vi "FTW-Example-SLASD-Launch.vi"(9 "Timeout":i32=1000 format="%dmsec", 11 "error in":errorcluster) -> (4 "FTW Actor Connector":refnum<class "FTW-Example-SLASD.lvclass">, 6 "Initialized Response":string, 8 "Instance Inbox Address":string, 10 "Instance Publisher Address":string, 15 "error out":errorcluster)   [LabVIEW 2013]
uses:
  FTW-Example-SLASD.lvclass
  Actor/src/Connector/FTW-ActorConnector.lvclass
  Core/FTW-Example-SLASD-Core.lvclass
panel:
  in  "Boolean":bool
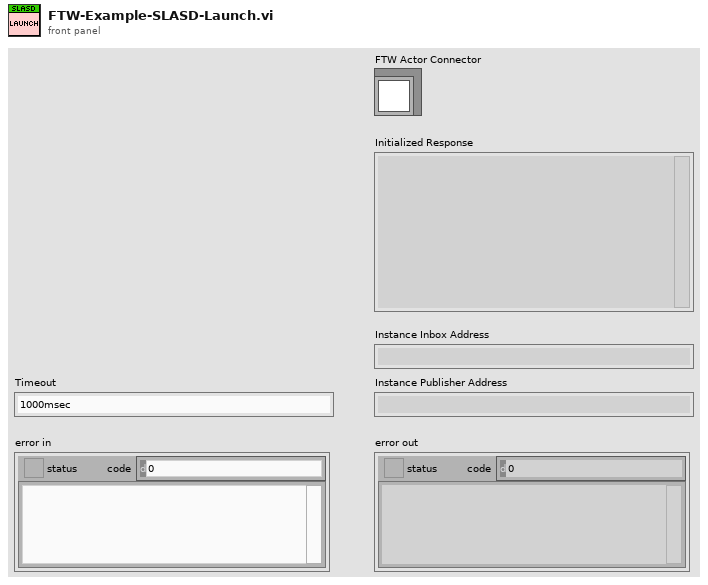
[diagram p1: front panel]
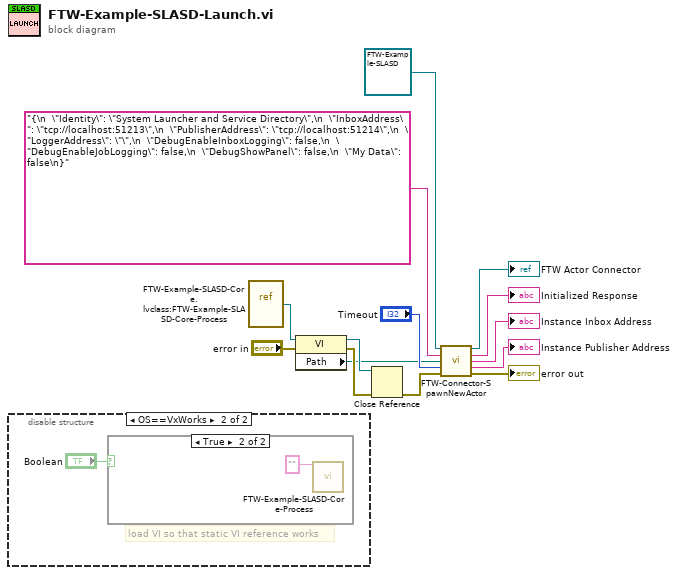
[diagram p0: block diagram]
diagram:
  n1 = disable-structure shown="OS==VxWorks" {
    frame condition #0 (active) {
    }
    frame condition #1 {
      # "load VI so that static VI reference works"
      n2 = case shown="True" "Boolean" {
        frame False {
        }
        frame True {
          n3 = call "FTW-Example-SLASD-Core-Process.vi"(0:"" ("FTW Actor Instance Configuration")) -> ()  [unwired: 15 in]
        }
      }
    }
  }
  n4 = vi-ref "FTW-Example-SLASD-Core.lvclass:FTW-Example-SLASD-Core-Process.vi"() -> (w6:refnum<vi>)
  n5 = property class="VI"(reference=w6, error in="error in") -> (reference out=w5:refnum<vi>, error out=w4:errorcluster, "Path"=w1:path)
  n6 = Close Reference(reference=w5, error in (no error)=w4) -> (error out=w2:errorcluster)
  n7 = call "FTW-Connector-SpawnNewActor.vi"("FTW Actor Connector Type"=refnum<class "FTW-Example-SLASD.lvclass"> refnum ("TTK_Splashscreen.lvclass"), "Configuration"="{\n  \"Identity\": \"System Launcher and Service Directory\",\n  \"InboxAddress\": \"tcp://localhost:51213\",\n  \"PublisherAddress\": \"tcp://localhost:51214\",\n  \"LoggerAddress\": \"\",\n  \"DebugEnableInboxLogging\": false,\n  \"DebugEnableJobLogging\": false,\n  \"DebugShowPanel\": false,\n  \"My Data\": false\n}", "Actor VI Filepath"=w1, "Timeout"="Timeout", "error in"=w2) -> ("FTW Actor Connector"=→"FTW Actor Connector":refnum<class "FTW-Example-SLASD.lvclass">, "Initialized Response"=→"Initialized Response":string, "Instance Inbox Address"=→"Instance Inbox Address":string, "Instance Publisher Address"=→"Instance Publisher Address":string, "error out"=→"error out":errorcluster)  [unwired: 6 in]
